vi "MoveCrd.vi"(6 "Dinstance Multiplier":i32=40, 8 "error in":errorcluster, 9 "FinalY":dbl, 10 "FinalX":dbl, 11 "Current Crd":refnum<vi>[](array[refnum])) -> (0 "error out":errorcluster)   [LabVIEW 2021]
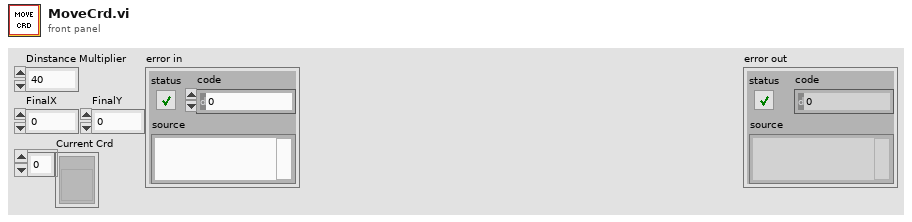
[diagram p1: front panel]
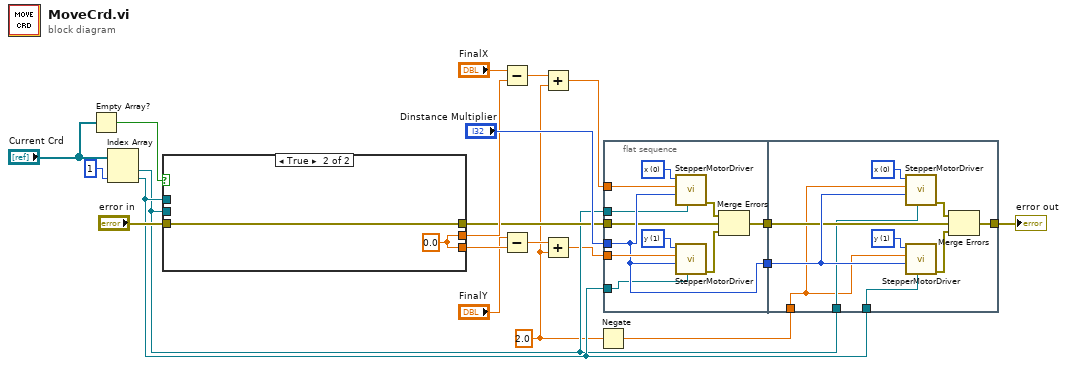
[diagram p0: block diagram]
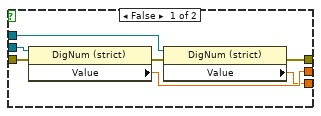
[diagram p2: hidden frame]
diagram:
  w2 = 2.0 ("y")
  n1 = Empty Array?(array="Current Crd") -> (empty?=w7:bool)
  n2 = Index Array(array="Current Crd", index #2=1 ("index")) -> (element #1=w8:refnum<vi>, element #2=w10:refnum<vi>)  [unwired: 1 in]
  n3 = case shown="True" w7 {
    tunnel: [w28 w30] -> w17
    tunnel: [w27 w30] -> w16
    tunnel: "error in" -> [w26 w29]
    tunnel: [w24 w29] -> w12
    tunnel: w10 -> [w23 _]
    tunnel: w8 -> [w22 _]
    frame False {
      n4 = property class="DigNum (strict)"(reference=w22, error in=w26) -> (error out=w25:errorcluster, "Value"=w28:dbl)  [unwired: 1 out]
      n5 = property class="DigNum (strict)"(reference=w23, error in=w25) -> (error out=w24:errorcluster, "Value"=w27:dbl)  [unwired: 1 out]
    }
    frame True {
      w30 = 0.0 ("Value")
    }
  }
  n6 = Subtract(x="FinalX", y=w17) -> (x-y=w3:dbl)
  n7 = Subtract(x="FinalY", y=w16) -> (x-y=w6:dbl)
  n8 = Add(x=w3, y=w2) -> (x+y=w4:dbl)
  n9 = Add(x=w6, y=w2) -> (x+y=w5:dbl)
  n10 = Negate(x=w2) -> (-x=w1:dbl)
  n11 = flat-sequence {
    tunnel: w5 -> [w39]
    tunnel: w4 -> [w38]
    tunnel: "Dinstance Multiplier" -> [w37]
    tunnel: [w37] -> w20
    tunnel: [w35] -> w19
    tunnel: w12 -> [w33]
    tunnel: w8 -> [w32]
    tunnel: w10 -> [w31]
    tunnel: w20 -> [w49]
    tunnel: w19 -> [w48]
    tunnel: [w47] -> w11
    tunnel: w8 -> [w46]
    tunnel: w10 -> [w45]
    tunnel: w1 -> [w42]
    frame #0 {
      w40 = u16 1 items=["x", "y"] ("Direction")
      w41 = u16 0 items=["x", "y"] ("Direction")
      n12 = call "StepperMotorDriver.vi"("pCoordinate"=w32, "Dinstance Multiplier"=w37, "Distance"=w38, "Direction"=w41) -> ("error out"=w34:errorcluster)  [unwired: 7 in]
      n13 = call "StepperMotorDriver.vi"("pCoordinate"=w31, "Dinstance Multiplier"=w37, "Distance"=w39, "Direction"=w40) -> ("error out"=w36:errorcluster)  [unwired: 7 in]
      n14 = Merge Errors(w34, w33, w36) -> (w35:errorcluster)
    }
    frame #1 {
      w50 = u16 0 items=["x", "y"] ("Direction")
      w51 = u16 1 items=["x", "y"] ("Direction")
      n15 = call "StepperMotorDriver.vi"("pCoordinate"=w46, "Dinstance Multiplier"=w49, "Distance"=w42, "Direction"=w50) -> ("error out"=w44:errorcluster)  [unwired: 7 in]
      n16 = call "StepperMotorDriver.vi"("pCoordinate"=w45, "Dinstance Multiplier"=w49, "Distance"=w42, "Direction"=w51) -> ("error out"=w43:errorcluster)  [unwired: 7 in]
      n17 = Merge Errors(w44, w48, w43) -> (w47:errorcluster)
    }
  }
  "error out" <- w11
